vi "from string.vi"(8 "error in":errorcluster, 9 "data":string, 10 "version":string, 11 "fixed channel configuration in":refnum<class "fixed channel configuration.lvclass">) -> (0 "error out":errorcluster, 3 "fixed channel configuration out":refnum<class "fixed channel configuration.lvclass">)   [LabVIEW 2013, in "fixed channel configuration.lvclass"]
doc: "Provides an interface for loading a module configuration from a file or other serialized data source. It is recommended that all children of this class store data in two sets--data required for its own initialization, and any data required for parent initialization--and that each implementation uses the <b>Call Parent Method</b> primitive to de-serialize parent information. As a result, it is expected that every module configuration class calls <b>component configuration.lvclass:From String.vi</b>.\nNI Tag Bus Module Framework 1.0.3.43\nNI Systems Engineering"
uses:
  fixed channel configuration.lvclass
  <vilib>/NI/DCAF/Tag Editor Core/control module/configuration/control module configuration.lvclass
  <vilib>/NI/Tag Bus Module Framework/module configuration/TBM module configuration.lvclass
  <vilib>/NI/Configuration Framework/serializable configuration/NISE_CEF_serializable configuration.lvclass
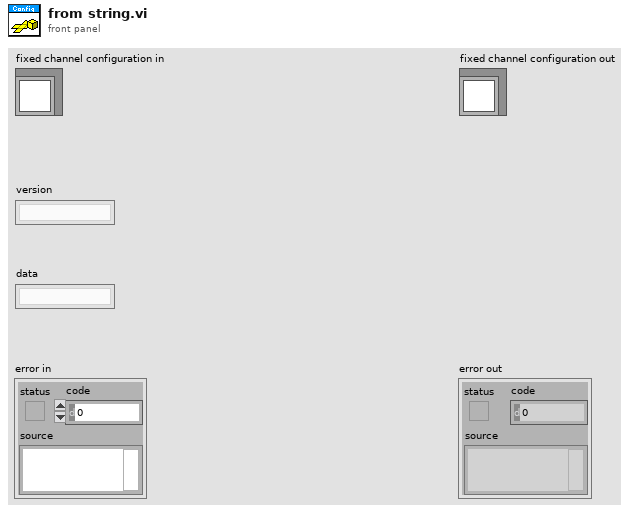
[diagram p1: front panel]
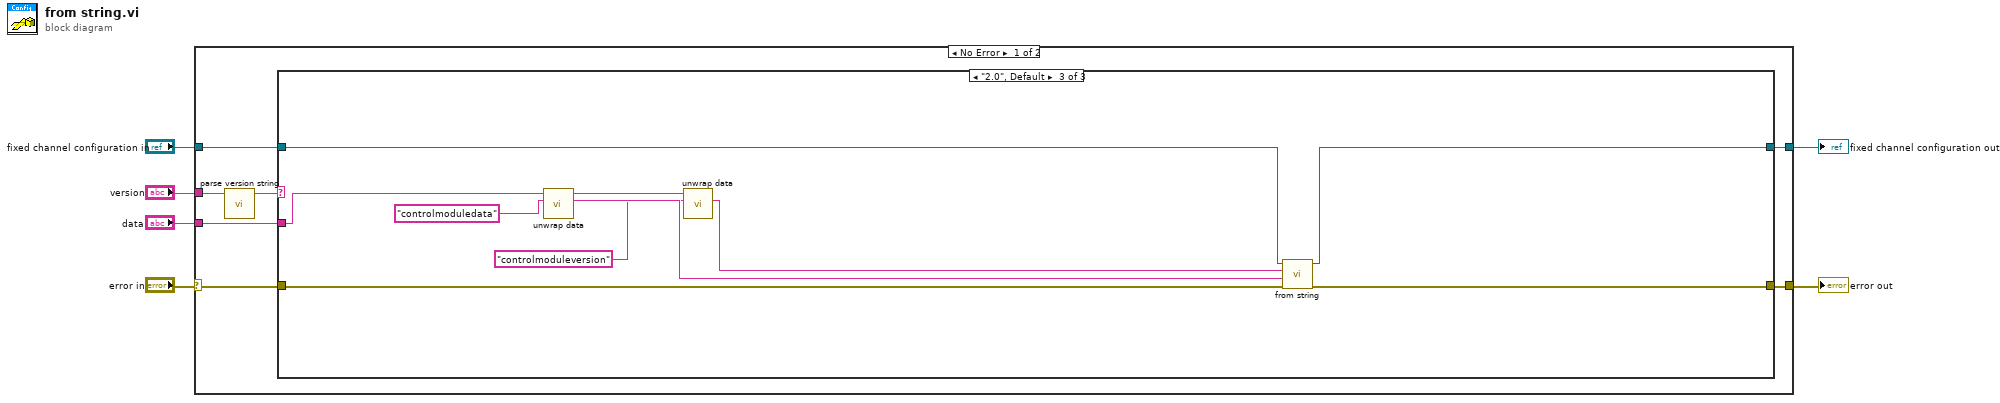
[diagram p0: block diagram]
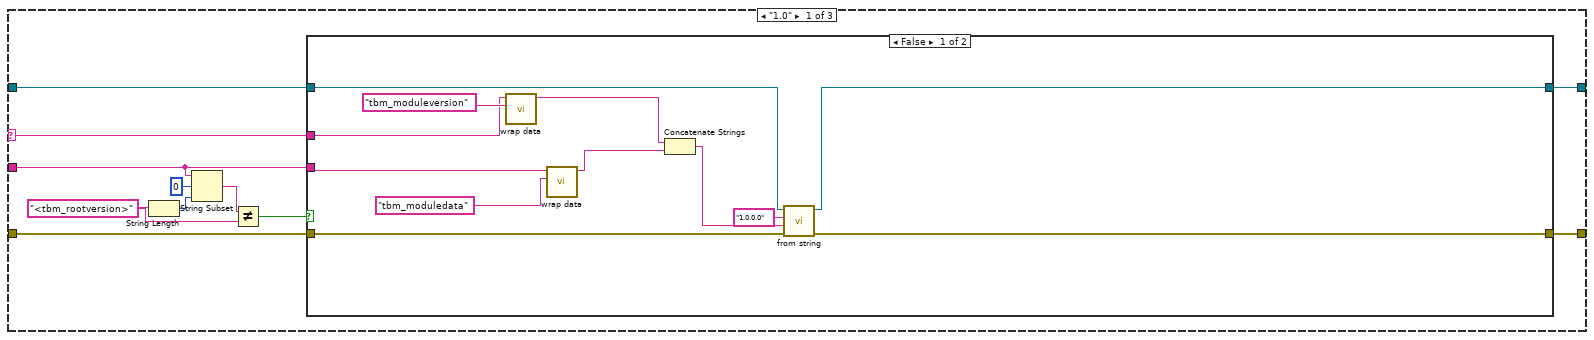
[diagram p2: hidden frame]
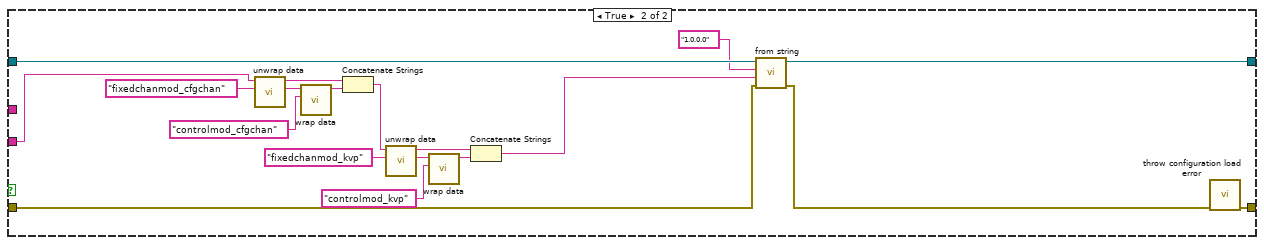
[diagram p3: hidden frame]
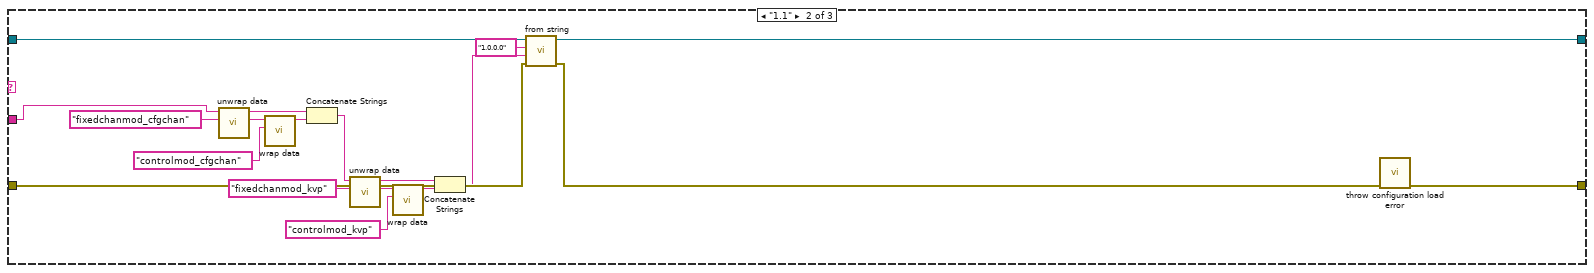
[diagram p4: hidden frame]
diagram:
  n1 = case shown="No Error" "error in" {
    selector: "error in" -> [w7 w86]
    tunnel: "data" -> [w13 _]
    tunnel: "fixed channel configuration in" -> [w12 w85]
    tunnel: [w11 w85] -> w5
    tunnel: [w10 w86] -> w4
    tunnel: "version" -> [w9 _]
    frame No Error {
      n2 = call <vilib>:"parse version string.vi"("full version"=w9) -> ("major.minor version"=w8:string)  [unwired: 7 in, 3 out]
      n3 = case shown="\"2.0\", Default" w8 {
        selector: w8 -> [w14 _ _]
        tunnel: w13 -> [w20 w57 w75]
        tunnel: w7 -> [w22 w72 w78]
        tunnel: w12 -> [w24 w74 w82]
        tunnel: [w21 w70 w83] -> w11
        tunnel: [w23 w73 w84] -> w10
        frame "1.0" {
          w18 = "<tbm_rootversion>"
          n4 = String Length(string=w18) -> (length=w19:i32)
          n5 = String Subset(string=w20, offset (0)=0, length (rest)=w19) -> (substring=w17:string)
          n6 = Not Equal?(x=w17, y=w18) -> (x != y?=w16:bool)
          n7 = case shown="False" w16 {
            tunnel: w24 -> [w35 w55]
            tunnel: [w33 w54] -> w23
            tunnel: w22 -> [w36 w53]
            tunnel: [w34 w51] -> w21
            tunnel: w20 -> [w29 w37]
            tunnel: w14 -> [w31 _]
            frame False {
              n8 = call <vilib>:"wrap data.vi"("identifier"="tbm_moduleversion" ("additional identifier"), "data to wrap"=w31) -> ("wrapped data"=w27:string)  [unwired: 9 in]
              n9 = call <vilib>:"wrap data.vi"("identifier"="tbm_moduledata" ("additional identifier"), "data to wrap"=w29) -> ("wrapped data"=w28:string)  [unwired: 9 in]
              n10 = Concatenate Strings(w27, w28) -> (w26:string)
              n11 = call-parent "from string.vi"("error in"=w36, "data"=w26, "version"="1.0.0.0", "fixed channel configuration in"=w35) -> ("error out"=w33:errorcluster, "fixed channel configuration out"=w34:refnum<class "fixed channel configuration.lvclass">)  [unwired: 6 in]
            }
            frame True {
              n12 = call <vilib>:"unwrap data.vi"("identifier"="fixedchanmod_cfgchan", "data to unwrap"=w37) -> ("unwrapped data"=w49:string, "remaining string"=w48:string)  [unwired: 8 in]
              n13 = call <vilib>:"wrap data.vi"("identifier"="controlmod_cfgchan", "data to wrap"=w49) -> ("wrapped data"=w47:string)  [unwired: 9 in]
              n14 = Concatenate Strings(w48, w47) -> (w41:string)
              n15 = call <vilib>:"unwrap data.vi"("identifier"="fixedchanmod_kvp", "data to unwrap"=w41) -> ("unwrapped data"=w42:string, "remaining string"=w43:string)  [unwired: 8 in]
              n16 = call <vilib>:"wrap data.vi"("identifier"="controlmod_kvp", "data to wrap"=w42) -> ("wrapped data"=w44:string)  [unwired: 9 in]
              n17 = Concatenate Strings(w43, w44) -> (w38:string)
              n18 = call-parent "from string.vi"("error in"=w53, "data"=w38, "version"="1.0.0.0", "fixed channel configuration in"=w55) -> ("error out"=w52:errorcluster, "fixed channel configuration out"=w51:refnum<class "fixed channel configuration.lvclass">)  [unwired: 6 in]
              n19 = call <vilib>:"throw configuration load error.vi"("error in"=w52) -> ("error out"=w54:errorcluster)  [unwired: 10 in]
            }
          }
        }
        frame "1.1" {
          n20 = call <vilib>:"unwrap data.vi"("identifier"="fixedchanmod_cfgchan", "data to unwrap"=w57) -> ("unwrapped data"=w69:string, "remaining string"=w68:string)  [unwired: 8 in]
          n21 = call <vilib>:"wrap data.vi"("identifier"="controlmod_cfgchan", "data to wrap"=w69) -> ("wrapped data"=w67:string)  [unwired: 9 in]
          n22 = Concatenate Strings(w68, w67) -> (w61:string)
          n23 = call <vilib>:"unwrap data.vi"("identifier"="fixedchanmod_kvp", "data to unwrap"=w61) -> ("unwrapped data"=w62:string, "remaining string"=w63:string)  [unwired: 8 in]
          n24 = call <vilib>:"wrap data.vi"("identifier"="controlmod_kvp", "data to wrap"=w62) -> ("wrapped data"=w64:string)  [unwired: 9 in]
          n25 = Concatenate Strings(w63, w64) -> (w58:string)
          n26 = call-parent "from string.vi"("error in"=w72, "data"=w58, "version"="1.0.0.0", "fixed channel configuration in"=w74) -> ("error out"=w71:errorcluster, "fixed channel configuration out"=w70:refnum<class "fixed channel configuration.lvclass">)  [unwired: 6 in]
          n27 = call <vilib>:"throw configuration load error.vi"("error in"=w71) -> ("error out"=w73:errorcluster)  [unwired: 10 in]
        }
        frame "2.0", Default {
          n28 = call <vilib>:"unwrap data.vi"("identifier"="controlmoduledata", "data to unwrap"=w75) -> ("unwrapped data"=w80:string, "remaining string"=w81:string)  [unwired: 8 in]
          n29 = call <vilib>:"unwrap data.vi"("identifier"="controlmoduleversion", "data to unwrap"=w81) -> ("unwrapped data"=w79:string)  [unwired: 8 in, 1 out]
          n30 = call-parent "from string.vi"("error in"=w78, "data"=w80, "version"=w79, "fixed channel configuration in"=w82) -> ("error out"=w84:errorcluster, "fixed channel configuration out"=w83:refnum<class "fixed channel configuration.lvclass">)  [unwired: 6 in]
        }
      }
    }
    frame Error {
    }
  }
  "error out" <- w4
  "fixed channel configuration out" <- w5
